vi "Clamp AET Max_Vertical.vi"(6 "Edge Options":T1={"Edge Polarity"=0, "Kernel Size"=3, "Width"=3, "Minimum Edge Strength"=10.0, "Interpolation Type"=enum."Bilinear Fixed", "Data Processing Method"=enum."Average"} {"Edge Polarity" items=["All Edges", "Rising Edges", "Falling Edges"]; "Minimum Edge Strength" format="%.2f"; "Width" step=2; "Kernel Size" step=2}, 7 "Settings":T3={"Contrast"=40, "Filter width"=4, "Steepness"=2, "Subsampling Ratio"=5, "Show Search Area"=FALSE, "Show Search Lines"=FALSE, "Show Edges Found"=FALSE, "Show Result"=TRUE}, 8 "error in (no error)":errorcluster, 9 "Coordinate System":T5 {"Measurement System"."Axis Reference" items=["Direct", "Indirect"]; "Measurement System"."Angle (deg)" format="%.2f"; "Measurement System"."Origin"."Y" format="%.2f"; "Measurement System"."Origin"."X" format="%.2f"; "Reference System"."Axis Reference" items=["Direct", "Indirect"]; "Reference System"."Angle (deg)" format="%.2f"; "Reference System"."Origin"."Y" format="%.2f"; "Reference System"."Origin"."X" format="%.2f"}, 10 "Rectangle":T6 {"Rotation" format="%.2f"; "Left" scale=0.0..1024.0; "Right" scale=0.0..1024.0}, 11 "Image":T4) -> (0 "error out":errorcluster, 1 "Coordinate System (duplicate)":T5 {"Measurement System"."Axis Reference" items=["Direct", "Indirect"]; "Measurement System"."Angle (deg)" format="%.2f"; "Measurement System"."Origin"."Y" format="%.2f"; "Measurement System"."Origin"."X" format="%.2f"; "Reference System"."Axis Reference" items=["Direct", "Indirect"]; "Reference System"."Angle (deg)" format="%.2f"; "Reference System"."Origin"."Y" format="%.2f"; "Reference System"."Origin"."X" format="%.2f"}, 2 "Distance":sgl format="%.2f", 3 "Image Out":T4, 5 "Edge Coordinates":cluster{"X":sgl, "Y":sgl}[](array[cluster]) {"Y" format="%.2f"; "X" format="%.2f"})   [LabVIEW 2014]
doc: "Modified NI Vertical Max Clamp with Rake-3 which uses Advanced Edge Detection."
uses:
  <vilib>/vision/Image Controls.llb/IMAQ Image.ctl
  <vilib>/vision/Measure.llb/Edge Options.ctl
  <vilib>/vision/Measure.llb/Edge Polarity.ctl
  <vilib>/vision/NI_Vision_Development_Module.lvlib
panel:
  out "Elapsed time (ms)":u32
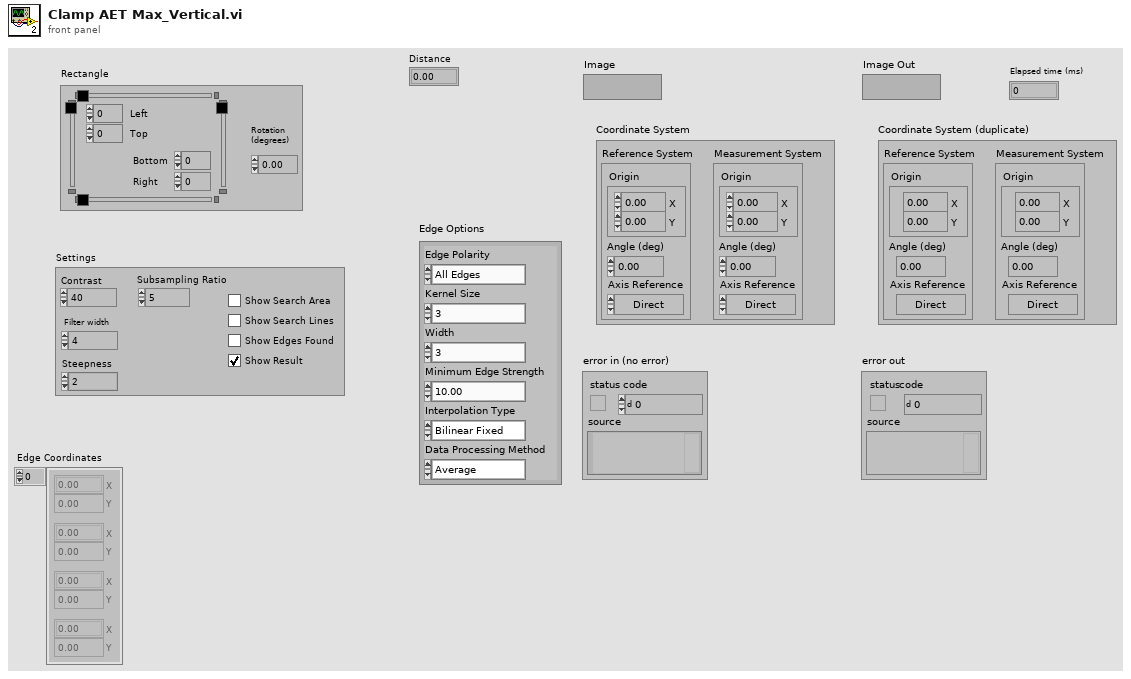
[diagram p1: front panel]
types:
  T1 = typedef "Edge Options.ctl" = cluster{"Edge Polarity":T2, "Kernel Size":u32, "Width":u32, "Minimum Edge Strength":sgl, "Interpolation Type":enum32{"Zero Order", "Bilinear", "Quadratic", "Cubic", "Bilinear Fixed"}, "Data Processing Method":enum32{"Average", "Median"}}
  T2 = typedef "Edge Polarity.ctl" = u32
  T3 = cluster{"Contrast":i32, "Filter width":i32, "Steepness":i32, "Subsampling Ratio":u32, "Show Search Area":bool, "Show Search Lines":bool, "Show Edges Found":bool, "Show Result":bool}
  T4 = typedef "IMAQ Image.ctl" = refnum<image>
  T5 = typedef "IMAQ Coordinate System" = cluster{"Reference System":cluster{"Origin":cluster{"X":sgl, "Y":sgl}, "Angle (deg)":sgl, "Axis Reference":u32}, "Measurement System":cluster{"Origin":cluster{"X":sgl, "Y":sgl}, "Angle (deg)":sgl, "Axis Reference":u32}}
  T6 = typedef "IMAQ Rectangle" = cluster{"Left":i32, "Top":i32, "Right":i32, "Bottom":i32, "Rotation":dbl}
  T7 = enum32{"Get First Edge", "Get First + Last Edge", "Get All Edges"}
  T8 = cluster{"Start Point":cluster{"X":sgl, "Y":sgl}, "End Point":cluster{"X":sgl, "Y":sgl}}
  T9 = typedef "ROI Descriptor" = cluster{"Global Rectangle":i32[], "Contours":cluster{"ID":enum32{"External", "Internal"}, "Type":u32, "Coordinates":i32[]}[]}
  T10 = typedef "Edge New.ctl" = cluster{"Location (Pixel)":cluster{"X":sgl, "Y":sgl}, "Location (Real-World)":cluster{"X":sgl, "Y":sgl}, "Distance (Pixel)":dbl, "Distance (Real-World)":dbl, "Strength":dbl, "Noise":dbl, "Rising?":bool}
  T11 = typedef "Search Line.ctl" = cluster{"Start Point":cluster{"X":sgl, "Y":sgl}, "End Point":cluster{"X":sgl, "Y":sgl}, "Edge Info":T10[], "Edge Map":dbl[], "Calibration Valid":bool}
  T12 = cluster{cluster{"X":sgl, "Y":sgl}, cluster{"X":sgl, "Y":sgl}}[]
  T13 = cluster{"Show Search Area":bool, "Show Search Lines":bool, "Show Edges Found":bool, "Show Result":bool}
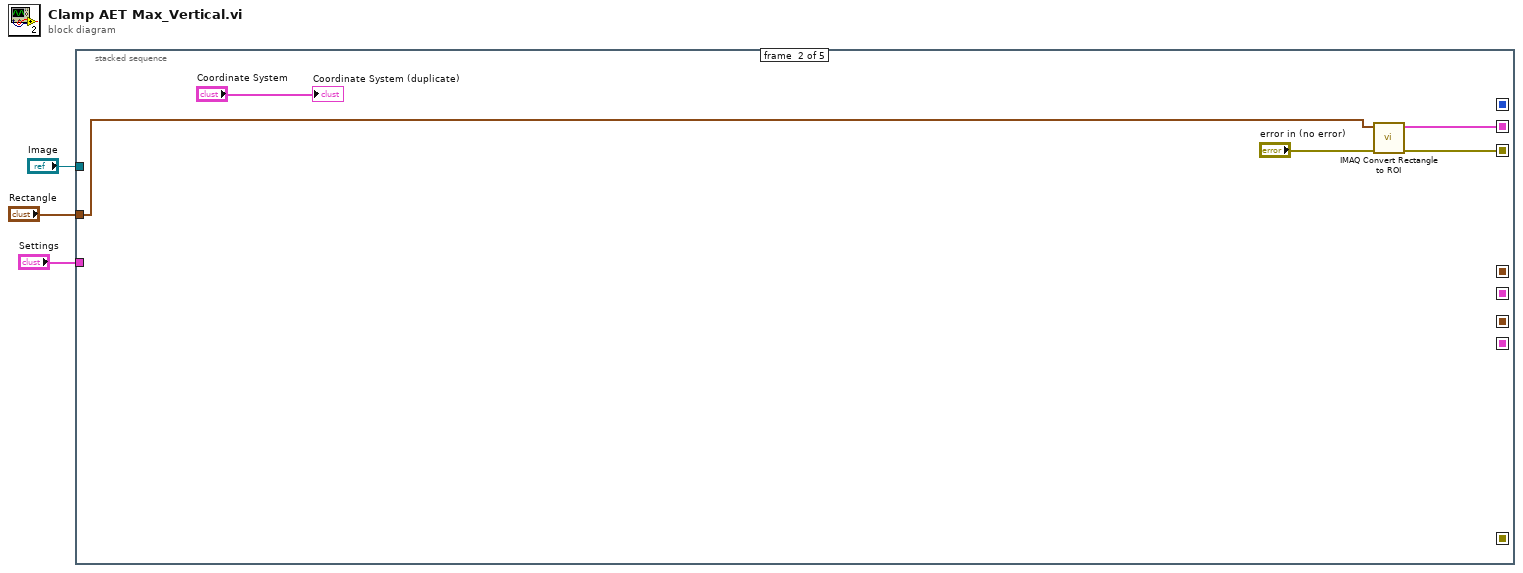
[diagram p0: block diagram]
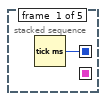
[diagram p2: hidden frame]
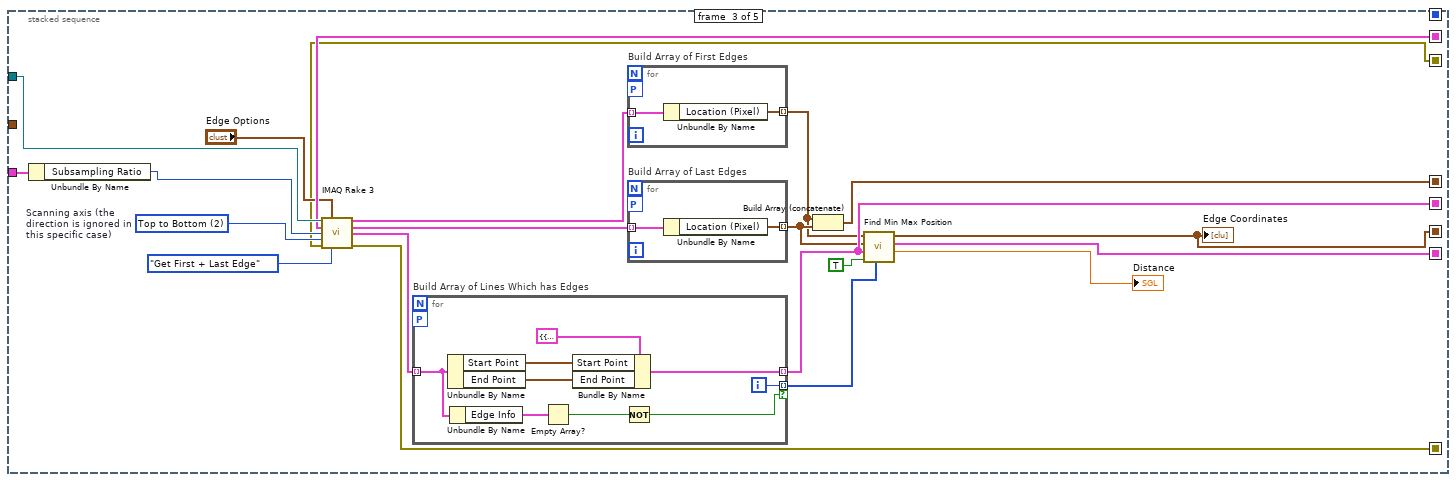
[diagram p3: hidden frame]
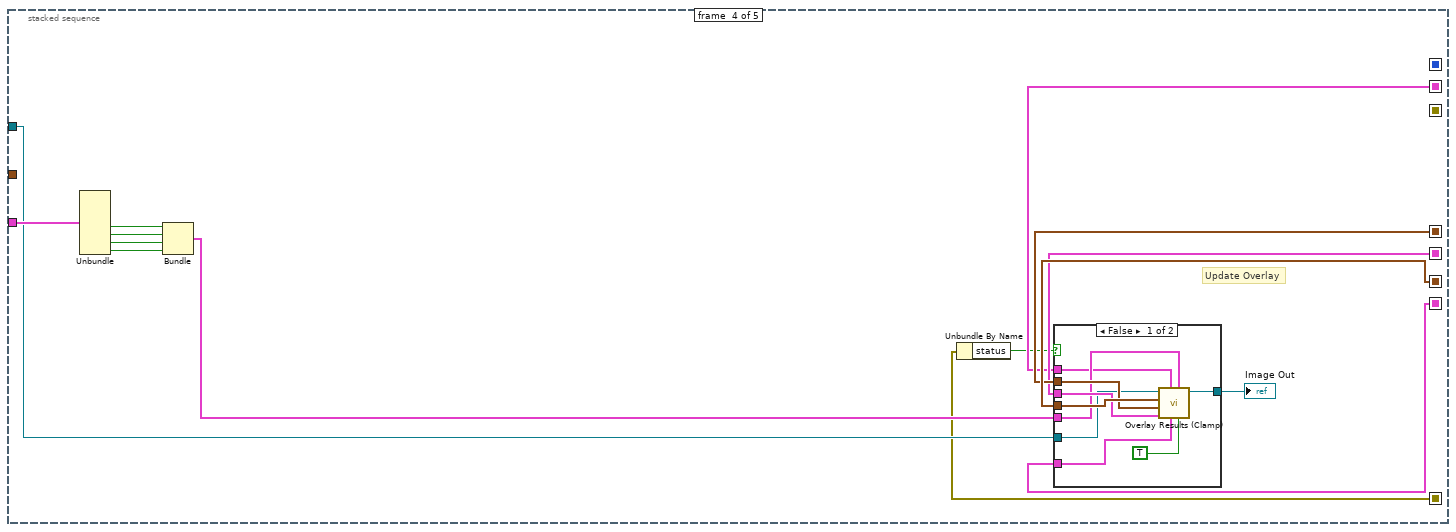
[diagram p4: hidden frame]
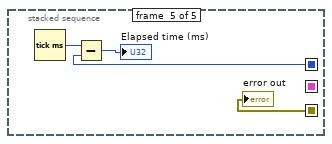
[diagram p6: hidden frame]
diagram:
  n1 = stacked-sequence {
    seq-local: [_ _ w16 _ _] -> [_ _ _ w58 _]
    seq-local: [w4 _ _ _ _] -> [_ _ _ _ w72]
    seq-local: [_ _ w18 _ _] -> [_ _ _ w57 _]
    seq-local: [_ _ w20 _ _] -> [_ _ _ w56 _]
    seq-local: [_ _ w17 _ _] -> [_ _ _ w50 _]
    seq-local: [_ w5 _ _ _] -> [_ _ w28 w48 _]
    seq-local: [_ w7 _ _ _] -> [_ _ w11 _ w69]
    seq-local: [_ _ w10 _ _] -> [_ _ _ w44 _]
    tunnel: "Image" -> [_ _ w29 w47 _]
    tunnel: "Rectangle" -> [_ w8 _ _ _]
    tunnel: "Settings" -> [_ _ w30 w55 _]
    frame #0 {
      n2 = Tick Count (ms)() -> (millisecond timer value=w4:u32)
    }
    frame #1 {
      n3 = call "IMAQ Convert Rectangle to ROI"("error in (no error)"="error in (no error)", "Rectangle"=w8) -> ("error out"=w7:errorcluster, "ROI Descriptor"=w5:T9)  [unwired: 7 out]
      "Coordinate System (duplicate)" <- "Coordinate System"
    }
    frame #2 {
      w26 = u32 2 items=["Left to Right", "Right to Left", "Top to Bottom", "Bottom to Top"]  # Scanning axis (the direction is ignored in this specific case)
      n4 = Unbundle By Name(w30) -> ("Subsampling Ratio"=w27:u32)
      n5 = call "IMAQ Rake 3"("Image"=w29, "Edge Options"="Edge Options", "ROI Descriptor"=w28, "Step Size"=w27, "Scan Direction"=w26, "error in (no error)"=w11, "Process"=T7."Get First + Last Edge") -> ("First Edges"=w23:T10[], "Last Edges"=w22:T10[], "Search Lines"=w21:T11[], "error out"=w10:errorcluster)  [unwired: 5 in]
      n6 = for "Build Array of Lines Which has Edges" {
        tunnel: w21 -> [w36] mode=indexing
        tunnel: [w37] -> w20 mode=indexing
        tunnel: [w33] -> w13 mode=indexing if=w32
        workers-P: _ -> [_]
        i -> [w33]
        n7 = Unbundle By Name(w36) -> ("Start Point"=w39:cluster{"X":sgl, "Y":sgl}, "End Point"=w38:cluster{"X":sgl, "Y":sgl})
        n8 = Unbundle By Name(w36) -> ("Edge Info"=w35:T10[])
        n9 = Empty Array?(array=w35) -> (empty?=w34:bool)
        n10 = Bundle By Name(cluster=T8 {"Start Point"={"X"=0.0, "Y"=0.0}, "End Point"={"X"=0.0, "Y"=0.0}} ("Cluster 2"), "Start Point"=w39, "End Point"=w38) -> (w37:T8)
        n11 = Not(x=w34) -> (.not. x?=w32:bool)
      }
      n12 = for "Build Array of First Edges" {
        tunnel: w23 -> [w43] mode=indexing
        tunnel: [w42] -> w14 mode=indexing
        workers-P: _ -> [_]
        n13 = Unbundle By Name(w43) -> ("Location (Pixel)"=w42:cluster{"X":sgl, "Y":sgl})
      }
      n14 = for "Build Array of Last Edges" {
        tunnel: w22 -> [w41] mode=indexing
        tunnel: [w40] -> w19 mode=indexing
        workers-P: _ -> [_]
        n15 = Unbundle By Name(w41) -> ("Location (Pixel)"=w40:cluster{"X":sgl, "Y":sgl})
      }
      n16 = Build Array (concatenate)(w14, w19) -> (w18:cluster{"X":sgl, "Y":sgl}[])
      n17 = call <vilib>:"Find Min Max Position.vi"("Lines with Edges (first)"=w13, "Min / Max"=TRUE, "Search Lines"=w20, "Last Edges"=w19, "First Edges"=w14) -> ("Distance"=→"Distance":sgl, "Perpendicular Lines"=w17:T12, "Points"=w16:cluster{"X":sgl, "Y":sgl}[])  [unwired: 1 in, 3 out]
      "Edge Coordinates" <- w16
    }
    frame #3 {
      # "Update Overlay"
      n18 = Unbundle(w55) -> ("Show Search Area"=w54:bool, "Show Search Lines"=w53:bool, "Show Edges Found"=w52:bool, "Show Result"=w51:bool)  [unwired: 4 out]
      n19 = Bundle("Show Search Area"=w54, "Show Search Lines"=w53, "Show Edges Found"=w52, "Show Result"=w51) -> (w49:T13)  [unwired: 1 out]
      n20 = Unbundle By Name(w44) -> ("status"=w45:bool)
      n21 = case shown="False" w45 {
        tunnel: w58 -> [w67 _]
        tunnel: w57 -> [w66 _]
        tunnel: w56 -> [w65 _]
        tunnel: w50 -> [w64 _]
        tunnel: w49 -> [w62 _]
        tunnel: w48 -> [w61 _]
        tunnel: w47 -> [w60 w68]
        tunnel: [w59 w68] -> w46
        frame False {
          n22 = call <vilib>:"Overlay Results (Clamp).vi"("Min / Max"=TRUE, "Setup"=w62, "Perpendicular Lines"=w64, "ROI Descriptor"=w61, "Search Lines"=w65, "All Edges Found"=w66, "Measurement Edges"=w67, "Image In"=w60) -> ("Image Out"=w59:T4)  [unwired: 3 out]
        }
        frame True {
        }
      }
      "Image Out" <- w46
    }
    frame #4 {
      n23 = Tick Count (ms)() -> (millisecond timer value=w71:u32)
      n24 = Subtract(x=w71, y=w72) -> (x-y=→"Elapsed time (ms)":u32)
      "error out" <- w69
    }
  }
